vi "Read Prober INI File.vi"(2 "configuration file path":path=path "C:/Users/Eddie.Rickey/Documents/RCV_PXI/Prober Configuration File.ini", 11 "Error In":errorcluster) -> (4 "Test Information":T1={"Exp Name"="Cold Switching", "Lot"="5khz_DC at 0V during Cycle_32V Land", "Wafer"="0233A", "Die Type"="15", "Die X "="L22", "Die Y"="6", "Exp"="8", "Die X_Y"="8"}, 6 "Start Test?":bool, 15 "Error Out":errorcluster)   [LabVIEW 2013]
uses:
  Controls/Test Information.ctl
  <vilib>/Utility/config.llb/Read Key (String).vi
  <vilib>/Utility/config.llb/NI_LVConfig.lvlib
panel:
  out "Test Complete?":bool
  out "Prober Ready?":string
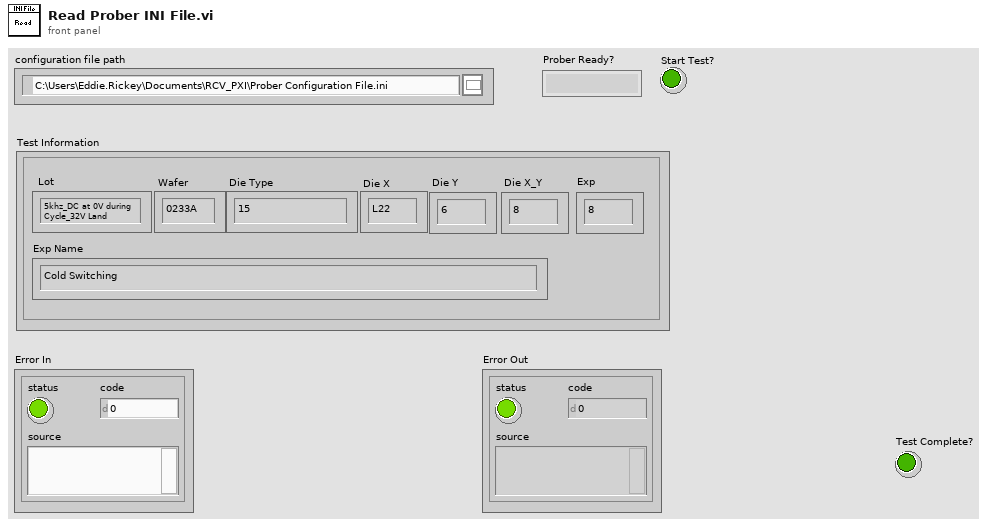
[diagram p1: front panel]
types:
  T1 = typedef "Test Information.ctl" = cluster{"Exp Name":string, "Lot":string, "Wafer":string, "Die Type":string, "Die X ":string, "Die Y":string, "Exp":string, "Die X_Y":string}
  T2 = typedef "NI_LVConfig.lvlib/Config Data RefNum.ctl" = refnum<k1>
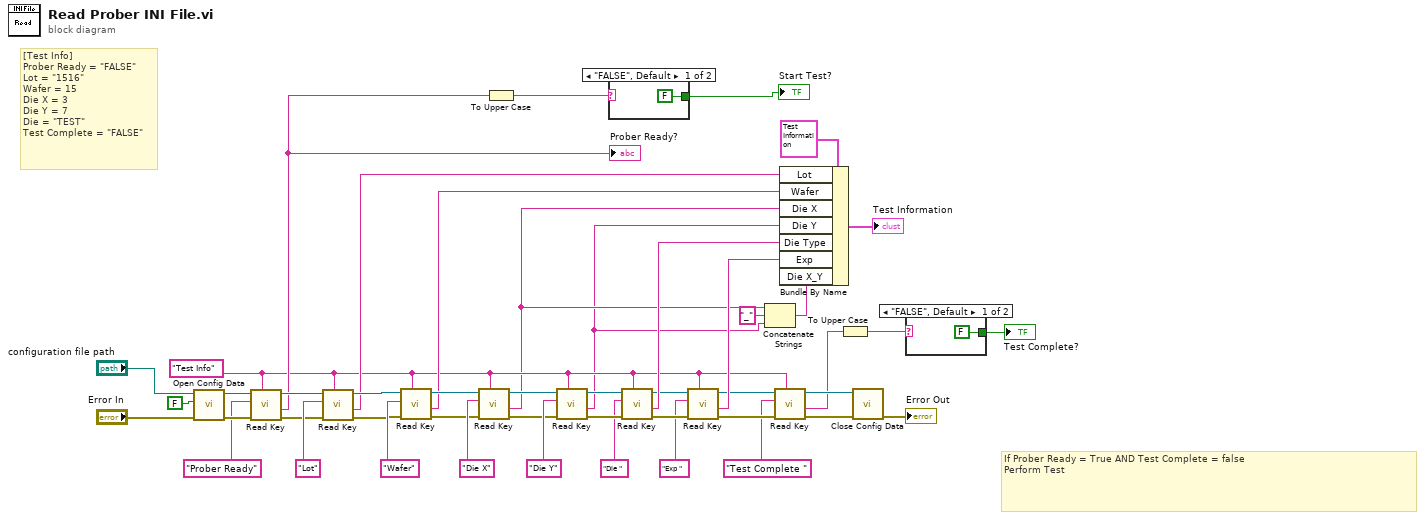
[diagram p0: block diagram]
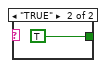
[diagram p2: hidden frame]
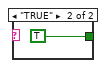
[diagram p3: hidden frame]
diagram:
  w10 = "Test Info" ("section")
  # "If Prober Ready = True AND Test Complete = false\nPerform Test"
  # "[Test Info]\nProber Ready = \"FALSE\"\nLot = \"1516\"\nWafer = 15\nDie X = 3\nDie Y = 7\nDie = \"TEST\"\nTest Complete = \"FALSE\""
  n1 = call <vilib>:"Open Config Data.vi"("error in (no error)"="Error In", "create file if necessary (T)"=FALSE, "configuration file path"="configuration file path") -> ("error out"=w46:errorcluster, "refnum"=w47:T2)  [unwired: 6 in, 1 out]
  n2 = call-poly <vilib>:"Read Key.vi"("section"=w10, "error in (no error)"=w46, "key"="Prober Ready", "refnum"=w47) -> ("error out"=w40:errorcluster, "value"=w16:string, "refnum out"=w41:T2)  [unwired: 4 in, 1 out]
  "Prober Ready?" <- w16
  n3 = call-poly <vilib>:"Read Key.vi"("section"=w10, "error in (no error)"=w40, "key"="Lot", "refnum"=w41) -> ("error out"=w38:errorcluster, "value"=w29:string, "refnum out"=w37:T2)  [unwired: 4 in, 1 out]
  n4 = call-poly <vilib>:"Read Key.vi"("section"=w10, "error in (no error)"=w38, "key"="Wafer", "refnum"=w37) -> ("error out"=w34:errorcluster, "value"=w28:string, "refnum out"=w33:T2)  [unwired: 4 in, 1 out]
  n5 = call-poly <vilib>:"Read Key.vi"("section"=w10, "error in (no error)"=w34, "key"="Die X", "refnum"=w33) -> ("error out"=w32:errorcluster, "value"=w4:string, "refnum out"=w31:T2)  [unwired: 4 in, 1 out]
  n6 = To Upper Case(1:w16) -> (0:w15:string)
  n7 = call-poly <vilib>:"Read Key.vi"("section"=w10, "error in (no error)"=w32, "key"="Die Y", "refnum"=w31) -> ("error out"=w23:errorcluster, "value"=w2:string, "refnum out"=w21:T2)  [unwired: 4 in, 1 out]
  n8 = case shown="\"FALSE\", Default" w15 {
    tunnel: [FALSE TRUE] -> w5
    frame "FALSE", Default {
    }
    frame "TRUE" {
    }
  }
  "Start Test?" <- w5
  n9 = call-poly <vilib>:"Read Key.vi"("section"=w10, "error in (no error)"=w23, "key"="Die ", "refnum"=w21) -> ("error out"=w24:errorcluster, "value"=w20:string, "refnum out"=w19:T2)  [unwired: 4 in, 1 out]
  n10 = call-poly <vilib>:"Read Key.vi"("section"=w10, "error in (no error)"=w24, "key"="Exp ", "refnum"=w19) -> ("error out"=w14:errorcluster, "value"=w17:string, "refnum out"=w11:T2)  [unwired: 4 in, 1 out]
  n11 = Concatenate Strings(w4, "_" ("string"), w2) -> (w1:string)
  n12 = call-poly <vilib>:"Read Key.vi"("section"=w10, "error in (no error)"=w14, "key"="Test Complete ", "refnum"=w11) -> ("error out"=w13:errorcluster, "value"=w7:string, "refnum out"=w12:T2)  [unwired: 4 in, 1 out]
  n13 = Bundle By Name(cluster=T1 {"Exp Name"="Cold Switching_Flat to Down", "Lot"="25khz Cycle Test_DC Measurement_PU Grounded", "Wafer"="1516", "Die Type"="14", "Die X "="Rbeam_1SC_CM1E", "Die Y"="6", "Exp"="8", "Die X_Y"=""} ("Test Information"), "Lot"=w29, "Wafer"=w28, "Die X"=w4, "Die Y"=w2, "Die Type"=w20, "Exp"=w17, "Die X_Y"=w1) -> (→"Test Information":T1)
  n14 = To Upper Case(1:w7) -> (0:w8:string)
  n15 = call <vilib>:"Close Config Data.vi"("error in (no error)"=w13, "refnum"=w12) -> ("error out"=→"Error Out":errorcluster)  [unwired: 8 in, 1 out]
  n16 = case shown="\"FALSE\", Default" w8 {
    tunnel: [FALSE TRUE] -> w6
    frame "FALSE", Default {
    }
    frame "TRUE" {
    }
  }
  "Test Complete?" <- w6
